vi "OceanDirectSample.vi"() -> ()   [LabVIEW 2021]
uses:
  C:/Program Files/Ocean Optics/OceanDirect SDK/lib/NetOceanDirect.dll
  Program Files/Ocean Optics/OceanDirect SDK/lib/NetOceanDirect.dll
panel:
  out "Spectrum":T1(graph)
  in  "?":bool
  in  "scansToAverage":u32
  in  "integrationTimeMicros":u32=100
  out "getApiVersion":dbl
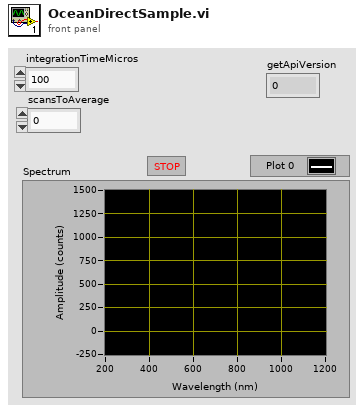
[diagram p1: front panel]
types:
  T1 = cluster{"getWavelengths":dbl[], "getSpectrum":dbl[]}
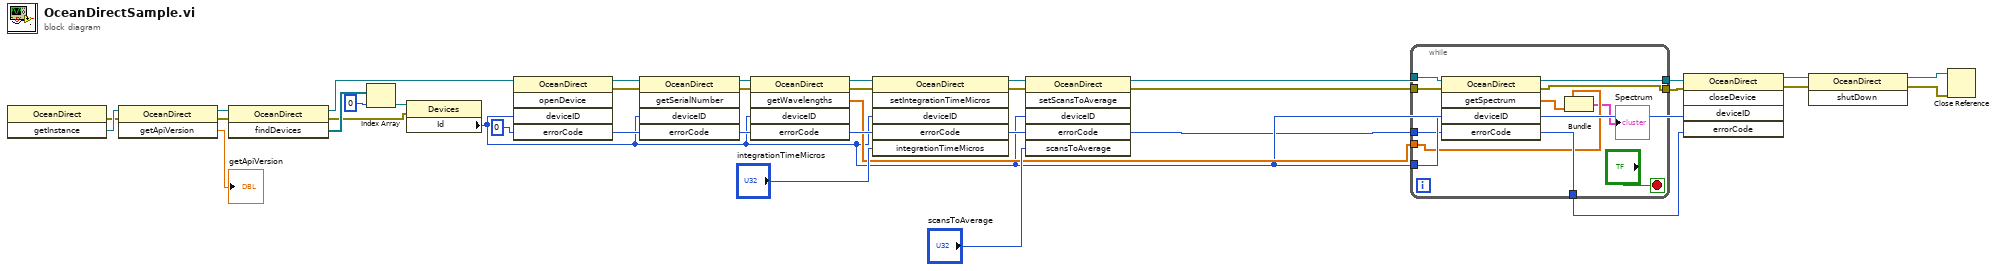
[diagram p0: block diagram]
diagram:
  n1 = invoke class="OceanDirect" method="getInstance"() -> (error out=w36:errorcluster, "getInstance"=w37:refnum<k24>)  [unwired: 3 in, 1 out]
  n2 = invoke class="OceanDirect" method="getApiVersion"(reference=w37, error in=w36) -> (reference out=w34:refnum<k24>, error out=w33:errorcluster, "getApiVersion"=→"getApiVersion":dbl)  [unwired: 1 in]
  n3 = invoke class="OceanDirect" method="findDevices"(reference=w34, error in=w33) -> (reference out=w29:refnum<k24>, error out=w30:errorcluster, "findDevices"=w32:refnum<k24>[])  [unwired: 1 in]
  n4 = Index Array(array=w32, index=0) -> (element=w31:refnum<k24>)
  n5 = property class="Devices"(reference=w31, error in=w30) -> ("Id"=w7:i32)  [unwired: 2 out]
  n6 = invoke class="OceanDirect" method="openDevice"(reference=w29, "deviceID"=w7, "errorCode"=0) -> (reference out=w26:refnum<k24>, error out=w25:errorcluster, "errorCode"=w18:i32)  [unwired: 2 in, 2 out]
  n7 = invoke class="OceanDirect" method="getSerialNumber"(reference=w26, error in=w25, "deviceID"=w7, "errorCode"=w18) -> (reference out=w24:refnum<k24>, error out=w23:errorcluster, "errorCode"=w17:i32)  [unwired: 1 in, 2 out]
  n8 = invoke class="OceanDirect" method="getWavelengths"(reference=w24, error in=w23, "deviceID"=w7, "errorCode"=w17) -> (reference out=w22:refnum<k24>, error out=w21:errorcluster, "getWavelengths"=w12:dbl[], "errorCode"=w16:i32)  [unwired: 1 in, 1 out]
  n9 = invoke class="OceanDirect" method="setIntegrationTimeMicros"(reference=w22, error in=w21, "deviceID"=w7, "errorCode"=w16, "integrationTimeMicros"="integrationTimeMicros") -> (reference out=w20:refnum<k24>, error out=w19:errorcluster, "errorCode"=w15:i32)  [unwired: 1 in, 3 out]
  n10 = invoke class="OceanDirect" method="setScansToAverage"(reference=w20, error in=w19, "deviceID"=w7, "errorCode"=w15, "scansToAverage"="scansToAverage") -> (reference out=w2:refnum<k24>, error out=w1:errorcluster, "errorCode"=w3:i32)  [unwired: 1 in, 3 out]
  n11 = while {
    tunnel: w2 -> [w48]
    tunnel: w1 -> [w47]
    tunnel: w7 -> [w46]
    tunnel: w3 -> [w45]
    tunnel: w12 -> [w39]
    tunnel: [w43] -> w11
    tunnel: [w42] -> w10
    tunnel: [w41] -> w6
    stop <- "?" stop-if-true
    n12 = invoke class="OceanDirect" method="getSpectrum"(reference=w48, error in=w47, "deviceID"=w46, "errorCode"=w45) -> (reference out=w43:refnum<k24>, error out=w42:errorcluster, "getSpectrum"=w40:dbl[], "errorCode"=w41:i32)  [unwired: 1 in, 1 out]
    n13 = Bundle("getWavelengths"=w39, "getSpectrum"=w40) -> (→"Spectrum":T1)  [unwired: 1 in]
  }
  n14 = invoke class="OceanDirect" method="closeDevice"(reference=w11, error in=w10, "deviceID"=w7, "errorCode"=w6) -> (reference out=w9:refnum<k24>, error out=w8:errorcluster)  [unwired: 1 in, 3 out]
  n15 = invoke class="OceanDirect" method="shutDown"(reference=w9, error in=w8) -> (reference out=w5:refnum<k24>, error out=w4:errorcluster)  [unwired: 1 in, 1 out]
  n16 = Close Reference(reference=w5, error in (no error)=w4) -> ()  [unwired: 1 out]
